vi "Clear Trigger timer.vi"(8 "error in (no error)":errorcluster, 10 "Timer (1)":i32=1 min=1 max=4 step=1 format="%#.6g", 11 "VISA resource name":refnum<visa-resource-name>) -> (0 "error out":errorcluster, 3 "VISA resource name out":refnum<visa-resource-name>)   [LabVIEW 2018, in "Keithley 2450.lvlib"]
doc: "This VI clears the timer event detector and overrun indicator for the specified trigger timer number."
uses:
  <instrlib>/Keithley 2450/Keithley 2450.lvlib
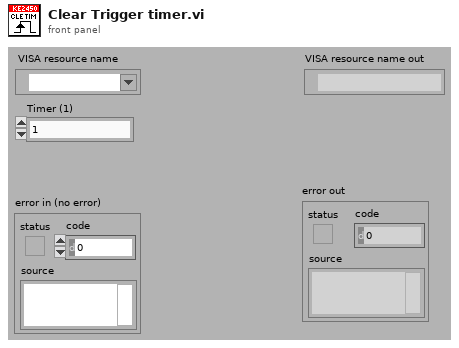
[diagram p1: front panel]
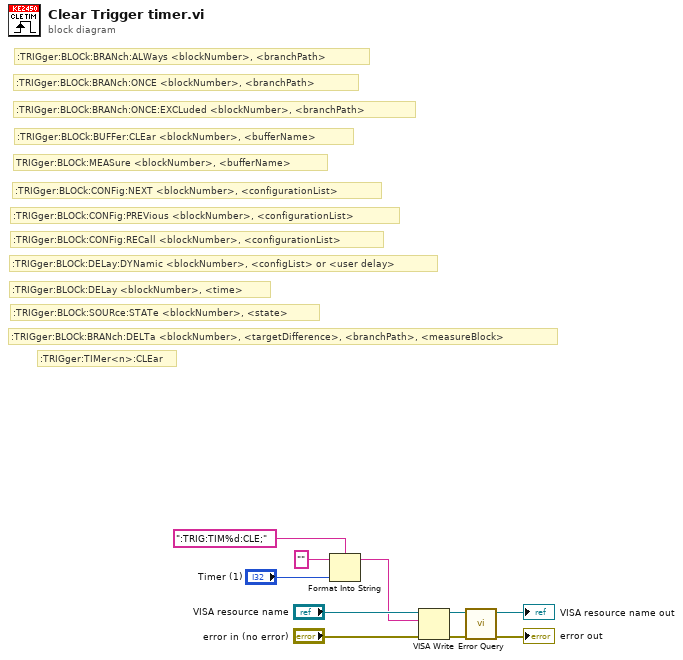
[diagram p0: block diagram]
diagram:
  # ":TRIGger:TIMer<n>:CLEar"
  # ":TRIGger:BLOCk:BRANch:DELTa <blockNumber>, <targetDifference>, <branchPath>, <measureBlock>"
  # ":TRIGger:BLOCk:SOURce:STATe <blockNumber>, <state>"
  # ":TRIGger:BLOCk:DELay <blockNumber>, <time>"
  # ":TRIGger:BLOCk:DELay:DYNamic <blockNumber>, <configList> or <user delay>"
  # ":TRIGger:BLOCk:CONFig:RECall <blockNumber>, <configurationList>"
  # ":TRIGger:BLOCk:CONFig:PREVious <blockNumber>, <configurationList>"
  # ":TRIGger:BLOCk:CONFig:NEXT <blockNumber>, <configurationList>"
  # "TRIGger:BLOCk:MEASure <blockNumber>, <bufferName>"
  # ":TRIGger:BLOCk:BUFFer:CLEar <blockNumber>, <bufferName>"
  # ":TRIGger:BLOCk:BRANch:ONCE:EXCLuded <blockNumber>, <branchPath>"
  # ":TRIGger:BLOCk:BRANch:ONCE <blockNumber>, <branchPath>"
  # ":TRIGger:BLOCk:BRANch:ALWays <blockNumber>, <branchPath>"
  n1 = Format Into String(format string=":TRIG:TIM%d:CLE;", initial string="", "Timer (1)") -> (resulting string=w1:string)  [unwired: 1 in, 1 out]
  n2 = VISA Write(VISA resource name="VISA resource name", write buffer=w1, error in (no error)="error in (no error)") -> (VISA resource name out=w6:refnum<visa-resource-name>, error out=w5:errorcluster)  [unwired: 1 out]
  n3 = call <instrlib>:"Error Query.vi"("error in (no error)"=w5, "VISA resource name"=w6) -> ("error out"=→"error out":errorcluster, "VISA resource name out"=→"VISA resource name out":refnum<visa-resource-name>)  [unwired: 8 out]
